vi "retrieveGoal.vi"(8 "error in (no error)":errorcluster, 10 "Goal.lvclass":refnum<class "Goal.lvclass">, 11 "Account History in":refnum<class "Account History.lvclass">) -> (0 "error out":errorcluster, 2 "Goal.lvclass":refnum<class "Goal.lvclass">, 3 "Account History out":refnum<class "Account History.lvclass">)   [LabVIEW 2018, in "Account History.lvclass"]
uses:
  Account History.lvclass
  Goal/Goal.lvclass
  C:/GitRepos/Filthy-Lucre-Budgetizer/source/support/classes/Category/Category.lvclass
  Category/Category.lvclass
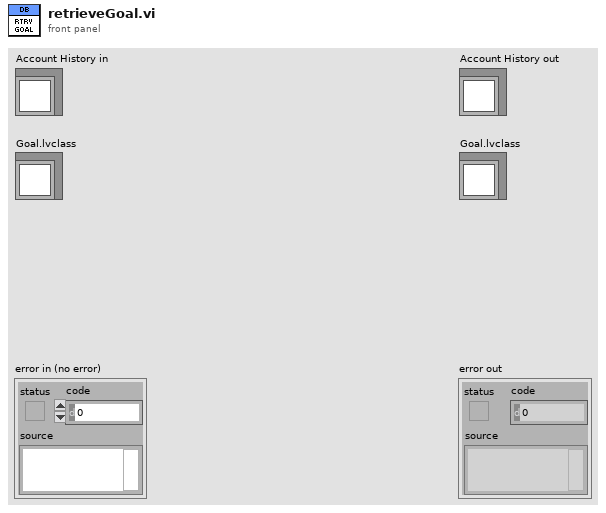
[diagram p1: front panel]
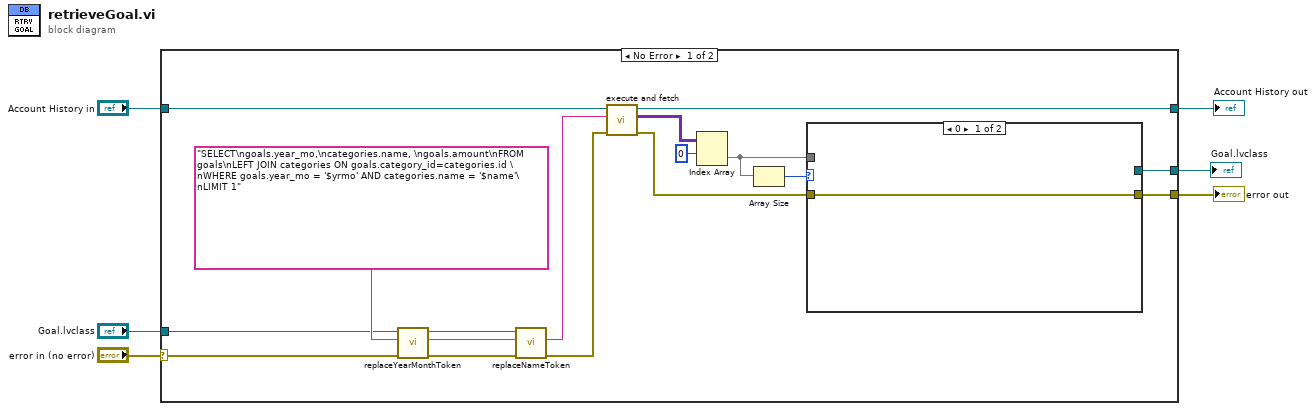
[diagram p0: block diagram]
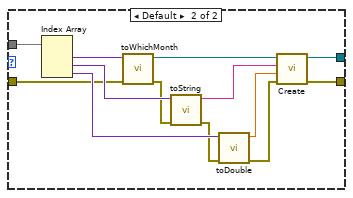
[diagram p2: hidden frame]
diagram:
  n1 = case shown="No Error" "error in (no error)" {
    selector: "error in (no error)" -> [w17 w39]
    tunnel: [w21 w39] -> w5
    tunnel: [w22 w38] -> w3
    tunnel: "Account History in" -> [w23 w38]
    tunnel: "Goal.lvclass" -> [w12 _]
    tunnel: [w7 _] -> w1
    frame No Error {
      n2 = call "replaceYearMonthToken.vi"("error in (no error)"=w17, "Querry In"="SELECT\ngoals.year_mo,\ncategories.name, \ngoals.amount\nFROM goals\nLEFT JOIN categories ON goals.category_id=categories.id \nWHERE goals.year_mo = '$yrmo' AND categories.name = '$name'\nLIMIT 1", "Goal in"=w12) -> ("error out"=w16:errorcluster, "Query Out"=w14:string, "Goal out"=w13:refnum<class "Goal.lvclass">)  [unwired: 6 in]
      n3 = call "replaceNameToken.vi"("error in (no error)"=w16, "Query In"=w14, "Category in"=w13) -> ("error out"=w18:errorcluster, "Query Out"=w19:string)  [unwired: 6 in, 1 out]
      n4 = call "execute and fetch.vi"("error in (no error)"=w18, "SQL query"=w19, "Database in"=w23) -> ("error out"=w20:errorcluster, "recordset data"=w10:variant[][], "Database out"=w22:refnum<class "Account History.lvclass">)  [unwired: 5 in, 1 out]
      n5 = Index Array(array=w10, index (row)=0) -> (element=w9:variant[])  [unwired: 1 in]
      n6 = Array Size(array=w9) -> (size(s)=w8:i32)
      n7 = case shown="0" w8 {
        tunnel: [w24 w26] -> w21
        tunnel: w20 -> [w24 w33]
        tunnel: w9 -> [_ w37]
        tunnel: [_ w25] -> w7
        frame 0 {
        }
        frame Default {
          n8 = Index Array(array=w37) -> (element #1=w35:variant, element #2=w34:variant, element #3=w36:variant)  [unwired: 3 in]
          n9 = call "toWhichMonth.vi"("error in (no error)"=w33, "Variant"=w35) -> ("error out"=w32:errorcluster, "WhichMonth.lvclass"=w30:refnum<class "WhichMonth.lvclass">)  [unwired: 8 in]
          n10 = call "toString.vi"("error in (no error)"=w32, "Variant"=w34) -> ("error out"=w31:errorcluster, "String"=w29:string)  [unwired: 8 in]
          n11 = call "toDouble.vi"("error in (no error)"=w31, "Value"=w36) -> ("error out"=w27:errorcluster, "type"=w28:dbl)  [unwired: 8 in]
          n12 = call "Create.vi"("error in (no error)"=w27, "Amount"=w28, "Category Name"=w29, "WhichMonth.lvclass"=w30) -> ("error out"=w26:errorcluster, "Goal out"=w25:refnum<class "Goal.lvclass">)  [unwired: 6 in]
        }
      }
    }
    frame Error {
    }
  }
  "error out" <- w5
  "Account History out" <- w3
  "Goal.lvclass" <- w1
